vi "Two Circles Optimization.vi"() -> ()   [LabVIEW 2023]
doc: "This example demonstrates how to use the Global Optimization VI to solve a multi-criteria optimization problem. The multi-criteria optimization problem can have multiple optima if objectives are well-defined or no optima if objectives conflict.\n\nThis example attempts to find a point that minimizes the distance between two circles simultaneously. A VI in the example implements the objective function, and a strictly typed reference of that VI is passed to the Global Optimization VI. All points between these two circles are the optima."
uses:
  <vilib>/gmath/GlobalOptimization.llb/DE_Settings.ctl
  <vilib>/gmath/GlobalOptimization.llb/DE_Bound Mapping Method.ctl
  <vilib>/gmath/GlobalOptimization.llb/DE_Mutation Method.ctl
  <vilib>/gmath/GlobalOptimization.llb/DE_Crossover Method.ctl
  <vilib>/gmath/GlobalOptimization.llb/DE_Stopping Criteria.ctl
  <vilib>/Analysis/1siggen.llb/Ramp Pattern by Samples.vi
  <vilib>/gmath/NI_AAL_GlobalOptimization.lvlib
  <vilib>/Analysis/NI_AALBase.lvlib
panel:
  in  "Population Size":i32=20 min=1 max=200 step=1
  out "number of optima":i32
  in  "Stop":bool
  out "Parameter Space":cluster{dbl[], dbl[]}[](graph)
  out "Objective Space":cluster{dbl[], dbl[]}(graph)
  # "Overview: Demonstrates multi-criteria optimization.\nRequirements: LabVIEW Full Development System\nInstructions:\n1. Run the VI. \n2. Observe the two graphs.\n3. Click Stop to stop the VI.\n4. Change the Population Size to 100 and run the VI again.\n3. Click Stop to stop the VI again."
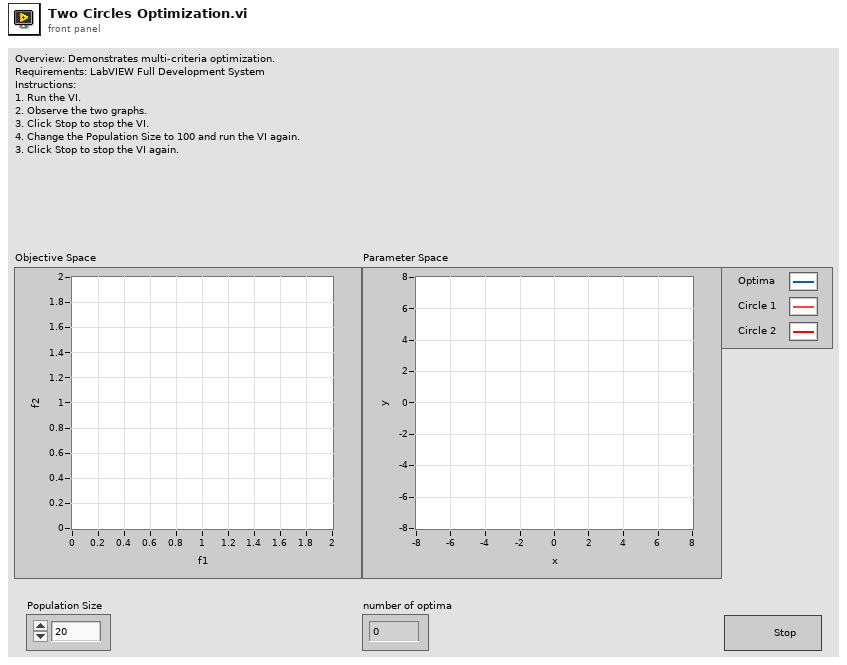
[diagram p1: front panel]
types:
  T1 = typedef "NI_AAL_GlobalOptimization.lvlib/DE_Stopping Criteria.ctl" = cluster{"max iterations":i32, "max function calls":i32, "max time (sec)":dbl}
  T2 = typedef "NI_AAL_GlobalOptimization.lvlib/DE_Settings.ctl" = cluster{"population size":i32, "scale factor":dbl, "crossover probability":dbl, "bound mapping method":T3, "mutation method":T4, "crossover method":T5}
  T3 = typedef "NI_AAL_GlobalOptimization.lvlib/DE_Bound Mapping Method.ctl" = u16
  T4 = typedef "NI_AAL_GlobalOptimization.lvlib/DE_Mutation Method.ctl" = u16
  T5 = typedef "NI_AAL_GlobalOptimization.lvlib/DE_Crossover Method.ctl" = u16
  T6 = typedef "NI_AAL_GlobalOptimization.lvlib/DE_State.ctl" = cluster{"Population":T7[], "Pareto Indexes":i32[]}
  T7 = typedef "NI_AAL_GlobalOptimization.lvlib/DE_Population.ctl" = cluster{"Parameters":dbl[], "Objective Functions":dbl[], "Equality Constraints":dbl[], "Inequality Constraints":dbl[]}
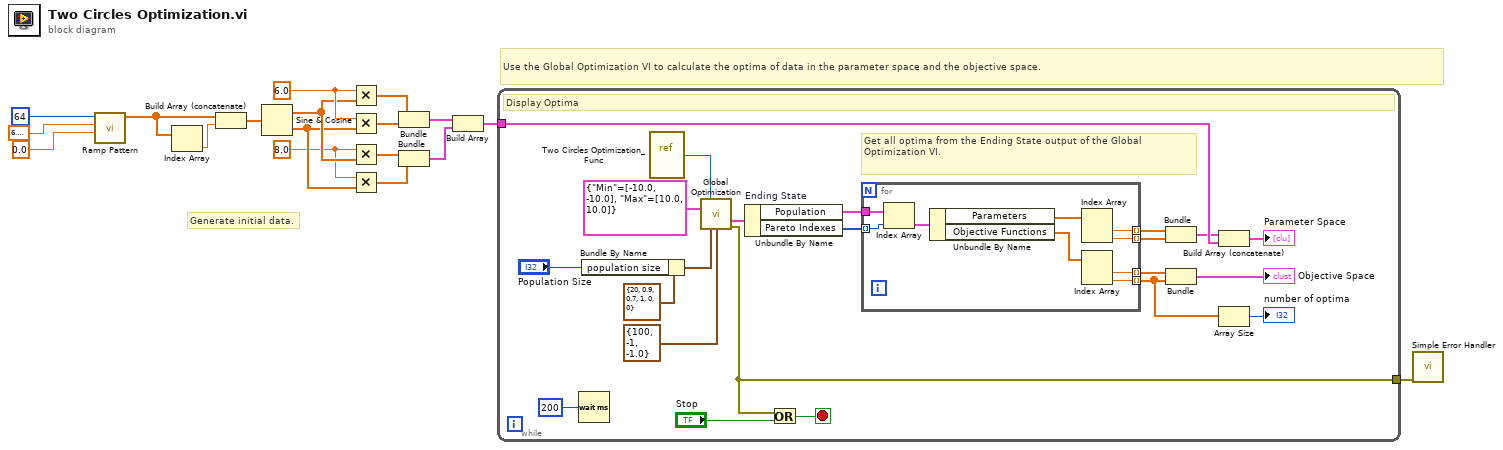
[diagram p0: block diagram]
diagram:
  w4 = 8.0
  w9 = 6.0
  # "Use the Global Optimization VI to calculate the optima of data in the parameter space and the objective space."
  # "Generate initial data."
  n1 = call-poly <vilib>:"Ramp Pattern.vi"("start"=0.0, "end"=6.283185307179586, "samples"=64) -> ("Ramp Pattern"=w14:dbl[])  [unwired: 7 in, 1 out]
  n2 = Index Array(array=w14) -> (element=w13:dbl)  [unwired: 1 in]
  n3 = Build Array (concatenate)(w14, w13) -> (w12:dbl[])
  n4 = Sine & Cosine(0:w12) -> (1:w6:dbl[], 2:w5:dbl[])
  n5 = Multiply(x=w9, y=w6) -> (x*y=w7:dbl[])
  n6 = Multiply(x=w9, y=w5) -> (x*y=w8:dbl[])
  n7 = Multiply(x=w4, y=w6) -> (x*y=w3:dbl[])
  n8 = Multiply(x=w4, y=w5) -> (x*y=w2:dbl[])
  n9 = Bundle(w7, w8) -> (w11:cluster{dbl[], dbl[]})  [unwired: 1 in]
  n10 = Bundle(w3, w2) -> (w10:cluster{dbl[], dbl[]})  [unwired: 1 in]
  n11 = Build Array(w11, w10) -> (w18:cluster{dbl[], dbl[]}[])
  n12 = while {
    tunnel: w18 -> [w34]
    tunnel: [w19] -> w1
    stop <- w20 stop-if-true
    # "Get all optima from the Ending State output of the Global Optimization VI."
    # "Display Optima"
    n13 = Wait (ms)(milliseconds to wait=u32 200) -> ()  [unwired: 1 out]
    n14 = Bundle By Name(cluster=T2 {"population size"=20, "scale factor"=0.9, "crossover probability"=0.7, "bound mapping method"=1, "mutation method"=0, "crossover method"=0} ("DE Settings"), "population size"="Population Size") -> (w23:T2)
    n15 = vi-ref "Two Circles Optimization_Func.vi"() -> (w40:refnum<vi>)
    n16 = call <vilib>:"Global Optimization.vi"("objective and constraint function"=w40, "Bounds"=cluster{"Min":dbl[], "Max":dbl[]} {"Min"=[-10.0, -10.0], "Max"=[10.0, 10.0]}, "DE settings"=w23, "stopping criteria"=T1 {"max iterations"=100, "max function calls"=-1, "max time (sec)"=-1.0}) -> ("Ending State"=w39:T6, "error out"=w19:errorcluster)  [unwired: 7 in, 3 out]
    n17 = Unbundle By Name "Ending State"(w39) -> ("Population"=w38:T7[], "Pareto Indexes"=w31:i32[])
    n18 = Or(x=w19, y="Stop") -> (x .or. y?=w20:bool)
    n19 = for {
      tunnel: w38 -> [w46]
      tunnel: [w48] -> w37 mode=indexing
      tunnel: [w47] -> w36 mode=indexing
      tunnel: w31 -> [w44] mode=indexing
      tunnel: [w42] -> w30 mode=indexing
      tunnel: [w41] -> w27 mode=indexing
      n20 = Index Array(array=w46, index=w44) -> (element=w45:T7)
      n21 = Unbundle By Name(w45) -> ("Parameters"=w49:dbl[], "Objective Functions"=w43:dbl[])
      n22 = Index Array(array=w49) -> (element #1=w48:dbl, element #2=w47:dbl)  [unwired: 2 in]
      n23 = Index Array(array=w43) -> (element #1=w42:dbl, element #2=w41:dbl)  [unwired: 2 in]
    }
    n24 = Bundle(w37, w36) -> (w33:cluster{dbl[], dbl[]})  [unwired: 1 in]
    n25 = Bundle(w30, w27) -> (→"Objective Space":cluster{dbl[], dbl[]})  [unwired: 1 in]
    n26 = Build Array (concatenate)(w33, w34) -> (→"Parameter Space":cluster{dbl[], dbl[]}[])
    n27 = Array Size(array=w27) -> (size(s)=→"number of optima":i32)
  }
  n28 = call <vilib>:"Simple Error Handler.vi"("error in (no error)"=w1) -> ()  [unwired: 4 in, 5 out]
